vi "Table_AllItems_Tests.vi"(8 "error in":errorcluster) -> (0 "error out":errorcluster)   [LabVIEW 2016, in "DronaTest.lvlib"]
uses:
  DronaTest.lvlib
  APIs/Stimulus/ControlValue/SetValueAuto.vi
  APIs/Stimulus/ControlValue/Controls/Table/SetValue.vi
  APIs/Assert/AssertControlValue/Controls/Table/AssertAllItems.vi
  <vilib>/addons/_JKI Toolkits/Caraya/classes/Assert/Assert Error.vi
  <vilib>/addons/_JKI Toolkits/Caraya/classes/Test/Test.lvclass
  <vilib>/SLL Toolkit/SLL Debug/SLL Debug.lvlib
  Drona.lvlib
  <vilib>/addons/_JKI Toolkits/Caraya/classes/Assert/Assert.lvclass
  APIs/Stimulus/ControlValue/ControlValue.lvlib
  APIs/Stimulus/ControlValue/Controls/Table/StimulusTable.lvlib
  APIs/Assert/AssertControlValue/Controls/Table/AssertTable.lvlib
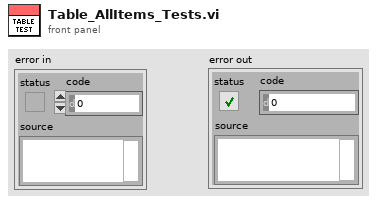
[diagram p1: front panel]
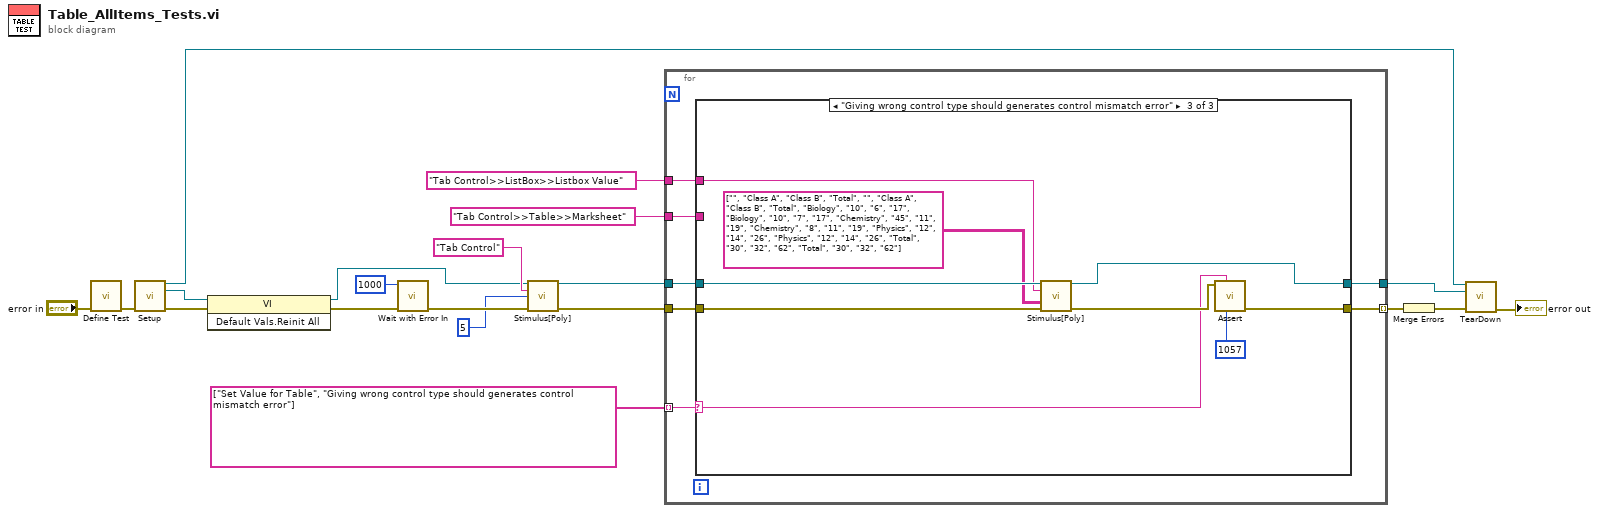
[diagram p0: block diagram]
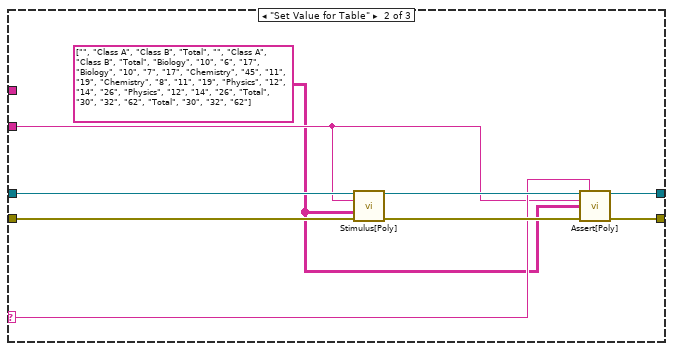
[diagram p3: hidden frame]
diagram:
  n1 = call <vilib>:"Define Test.vi"("error in (no error)"="error in") -> ("error out"=w10:errorcluster)  [unwired: 9 in, 1 out]
  n2 = call "Setup.vi"("error in (no error)"=w10) -> ("Application Ref"=w7:refnum<vi>, "VI out"=w2:refnum<vi>, "error out"=w9:errorcluster)  [unwired: 12 in]
  n3 = invoke class="VI" method="Default Vals.Reinit All"(reference=w2, error in=w9) -> (reference out=w1:refnum<vi>, error out=w3:errorcluster)  [unwired: 1 in, 1 out]
  n4 = call <vilib>:"Wait with Error In.vi"("error in (no error)"=w3, "milliseconds to wait"=u32 1000) -> ("error out"=w18:errorcluster)  [unwired: 9 in]
  n5 = call-poly "Stimulus[Poly].vi"("VI Reference In"=w1, "Control Path"="Tab Control", "Value (Signaling)"=5, "error in"=w18) -> ("VI Reference Out"=w14:refnum<vi>, "error out"=w17:errorcluster)  [unwired: 10 in]
  n6 = for {
    tunnel: w14 -> [w26]
    tunnel: "Tab Control>>Table>>Marksheet" ("Control Path") -> [w25]
    tunnel: "Tab Control>>ListBox>>Listbox Value" ("Control Path") -> [w24]
    tunnel: string[] ["Set Value for Table", "Giving wrong control type should generates control mismatch error"] -> [w22] mode=indexing
    tunnel: [w21] -> w6
    tunnel: w17 -> [w27]
    tunnel: [w23] -> w11 mode=indexing
    n7 = case shown="\"Giving wrong control type should generates control mismatch error\"" w22 {
      selector: w22 -> [_ w32 w43]
      tunnel: w27 -> [w29 w38 w47]
      tunnel: w26 -> [w28 w37 w46]
      tunnel: w25 -> [_ w31 _]
      tunnel: w24 -> [_ _ w40]
      tunnel: [w29 w34 w44] -> w23
      tunnel: [w28 w33 w41] -> w21
      frame Default {
      }
      frame "Set Value for Table" {
        w30 = string[][] [["", "Class A", "Class B", "Total", "", "Class A", "Class B", "Total"], ["Biology", "10", "6", "17", "Biology", "10", "7", "17"], ["Chemistry", "45", "11", "19", "Chemistry", "8", "11", "19"], ["Physics", "12", "14", "26", "Physics", "12", "14", "26"], ["Total", "30", "32", "62", "Total", "30", "32", "62"]] ("Value")
        n8 = call-poly "Stimulus[Poly].vi"("VI Reference In"=w37, "Control Path"=w31, "Value"=w30, "Error In"=w38) -> ("VI Reference Out"=w35:refnum<vi>, "Error Out"=w36:errorcluster)  [unwired: 10 in]
        n9 = call-poly "Assert[Poly].vi"("VI Reference In"=w35, "Test Label"=w32, "Control Path"=w31, "Item Value"=w30, "Error In"=w36) -> ("VI Reference Out"=w33:refnum<vi>, "Error Out"=w34:errorcluster)  [unwired: 8 in, 1 out]
      }
      frame "Giving wrong control type should generates control mismatch error" {
        n10 = call-poly "Stimulus[Poly].vi"("VI Reference In"=w46, "Control Path"=w40, "Value"=string[][] [["", "Class A", "Class B", "Total", "", "Class A", "Class B", "Total"], ["Biology", "10", "6", "17", "Biology", "10", "7", "17"], ["Chemistry", "45", "11", "19", "Chemistry", "8", "11", "19"], ["Physics", "12", "14", "26", "Physics", "12", "14", "26"], ["Total", "30", "32", "62", "Total", "30", "32", "62"]], "Error In"=w47) -> ("VI Reference Out"=w41:refnum<vi>, "Error Out"=w45:errorcluster)  [unwired: 10 in]
        n11 = call-poly <vilib>:"Assert.vi"("error code (1)"=1057, "Label"=w43, "Error?"=w45) -> ("error out"=w44:errorcluster)  [unwired: 7 in, 1 out]
      }
    }
  }
  n12 = Merge Errors(w11) -> (w8:errorcluster)
  n13 = call "TearDown.vi"("Application Ref"=w7, "VI in"=w6, "error in (no error)"=w8) -> ("error out"=→"error out":errorcluster)  [unwired: 12 in]
